vi "Write Mission Msg.vi"(8 "error in (no error)":errorcluster, 9 "MissionOp":T1, 10 "index":i32, 11 "Load Mission Message in":refnum<class "Load Mission Message.lvclass">) -> (0 "error out":errorcluster, 3 "Load Mission Message out":refnum<class "Load Mission Message.lvclass">)   [LabVIEW 2015, in "RDS Child Messages.lvlib" / "Load Mission Message.lvclass"]
uses:
  Load Mission Message.lvclass
  RDS Mission Controller Actor/MissionOp.ctl
  Load Mission Message.lvclass/Load Mission Message.ctl
  RDS Mission Controller Actor/RDS Mission Controller Actor.lvlib
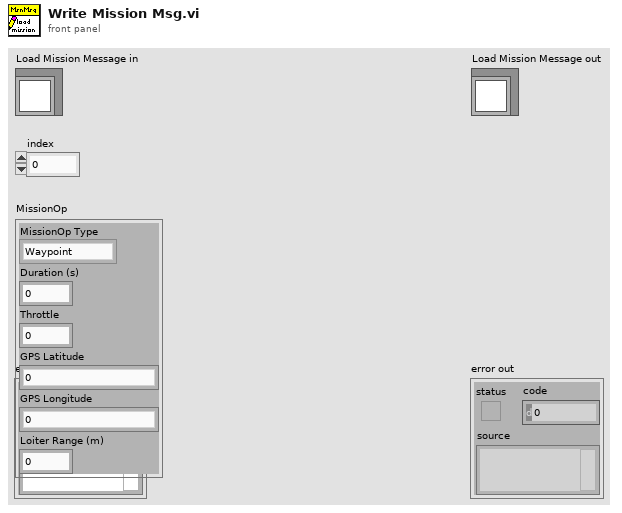
[diagram p1: front panel]
types:
  T1 = typedef "RDS Mission Controller Actor.lvlib/MissionOp.ctl" = cluster{"MissionOp Type":enum16{"Waypoint", "Loiter", "Wait", "Deploy AIP", "Stow AIP"}, "Duration (s)":dbl, "Throttle":dbl, "GPS Latitude":ext, "GPS Longitude":ext, "Loiter Range (m)":dbl}
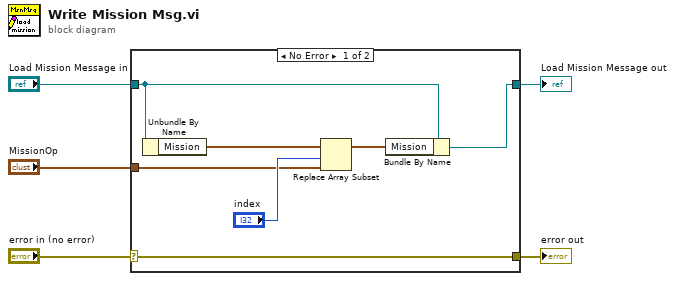
[diagram p0: block diagram]
diagram:
  n1 = case shown="No Error" "error in (no error)" {
    selector: "error in (no error)" -> [w12 w13]
    tunnel: [w12 w13] -> w4
    tunnel: [w11 w14] -> w2
    tunnel: "Load Mission Message in" -> [w10 w14]
    tunnel: "MissionOp" -> [w6 _]
    frame No Error {
      n2 = Unbundle By Name(w10) -> ("Mission"=w9:T1[])
      n3 = Replace Array Subset(array=w9, new element=w6, index="index") -> (w8:T1[])
      n4 = Bundle By Name(cluster=w10, "Mission"=w8) -> (w11:refnum<class "Load Mission Message.lvclass">)
    }
    frame Error {
    }
  }
  "error out" <- w4
  "Load Mission Message out" <- w2
